vi "test缓存测试.vi"() -> ()   [LabVIEW 2017, in "时值缓存压缩模块.lvlib"]
panel:
  out "等级数量":cluster{i32[], "压缩等级数量":i32[]}(graph)
  out "真起始时间":timestamp
  out "实际缓存数量":i32
  in  "停止按钮":bool
  out "大小":i32
  out "缓存处理用时":dbl
  out "缓存数据":cluster{"时间":timestamp[], "数值":dbl[]}(graph)
  in  "等待时间（毫秒）":u32=500
  in  "容量限值":i32=300 min=1
  in  "变化基数":dbl=3.0
  in  "主值":dbl=25.0 format="%#_13g"
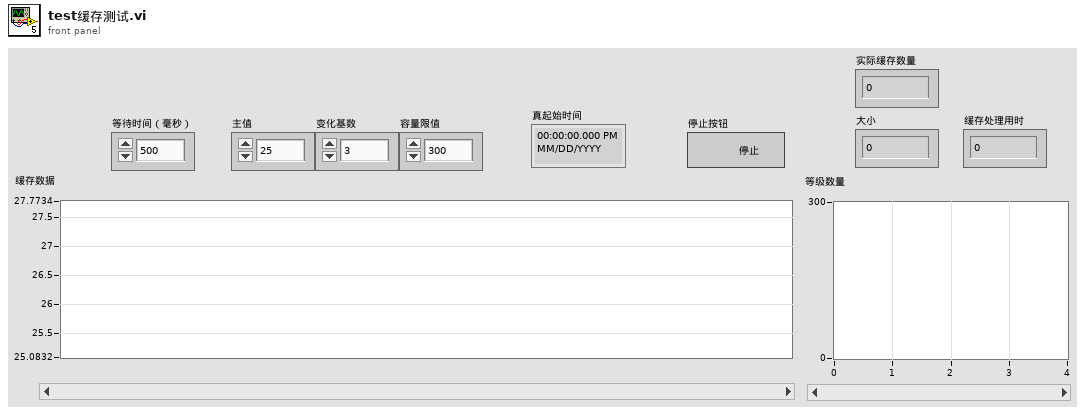
[diagram p1: front panel]
types:
  T1 = typedef "时值缓存压缩模块.lvlib/缓存数据.ctl" = cluster{"时间":timestamp[], "数值":dbl[], "压缩等级数量":i32[], "最大值":cluster{"时间":timestamp, "数值":dbl}, "起始点":cluster{"时间":timestamp, "数值":dbl}, "容量限值":i32, "报警累积":dbl}
  T2 = typedef "LVAnnotationListTypeDef.ctl" = cluster{"Name":string, "Color":u32, "Style":u8, "Point Style":u8, "Name Visible":bool, "Allow Drag":bool, "Annotation Mode":u32, "Plot":i32, "Index":i32, "Position":cluster{"X":dbl, "Y":dbl}, "X Scale":u32, "Y Scale":u32, "Show Arrow":bool, "Lock Name":bool, "Plot Area":i32, "Label Offset":cluster{"X":dbl, "Y":dbl}}[]
  T3 = cluster{"Name":string, "Color":u32, "Style":u8, "Point Style":u8, "Name Visible":bool, "Allow Drag":bool, "Annotation Mode":u32, "Plot":i32, "Index":i32, "Position":cluster{"X":dbl, "Y":dbl}, "X Scale":u32, "Y Scale":u32, "Show Arrow":bool, "Lock Name":bool, "Plot Area":i32, "Label Offset":cluster{"X":dbl, "Y":dbl}}
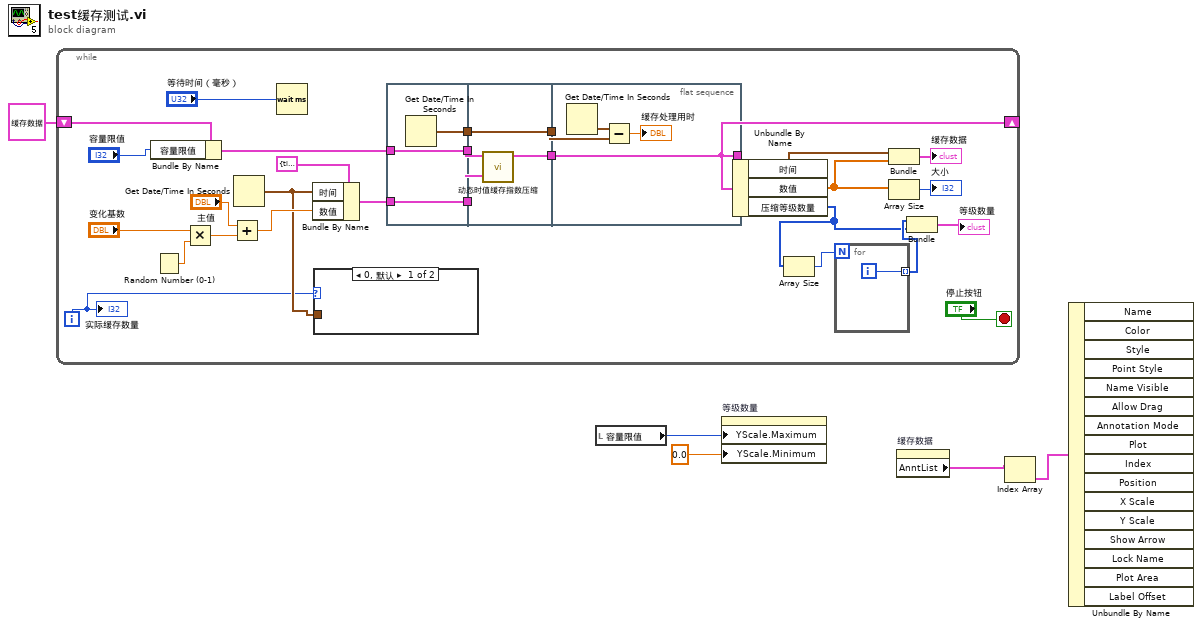
[diagram p0: block diagram]
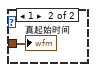
[diagram p2: hidden frame]
diagram:
  n1 = while {
    shift-right: [w22] -> _
    shift-left: T1 {"时间"=[], "数值"=[], "压缩等级数量"=[], "最大值"={"时间"=timestamp(0 s since 1904-01-01), "数值"=0.0}, "起始点"={"时间"=timestamp(0 s since 1904-01-01), "数值"=0.0}, "容量限值"=0, "报警累积"=0.0} ("缓存数据 i") -> [w26]
    i -> [w10]
    stop <- "停止按钮" stop-if-true
    n2 = Bundle By Name(cluster=w26, "容量限值"="容量限值") -> (w25:T1)
    n3 = Random Number (0-1)() -> (number: 0 to 1=w31:dbl)
    n4 = Multiply(x="变化基数", y=w31) -> (x*y=w32:dbl)
    n5 = Add(x="主值", y=w32) -> (x+y=w29:dbl)
    n6 = Get Date/Time In Seconds() -> (seconds since 1Jan1904=w11:timestamp)
    n7 = Wait (ms)(milliseconds to wait="等待时间（毫秒）") -> ()  [unwired: 1 out]
    n8 = Bundle By Name(cluster=cluster{"时间":timestamp, "数值":dbl} {"时间"=timestamp(0 s since 1904-01-01), "数值"=0.0} ("新数据"), "时间"=w11, "数值"=w29) -> (w27:cluster{"时间":timestamp, "数值":dbl})
    n9 = case shown="0, 默认" w10 {
      tunnel: w11 -> [_ w35]
      frame 0, Default {
      }
      frame 1 {
        "真起始时间" <- w35
      }
    }
    n10 = flat-sequence {
      tunnel: w25 -> [w37]
      tunnel: w27 -> [w38]
      tunnel: [w38] -> w19
      tunnel: [w37] -> w18
      tunnel: [w36] -> w16
      tunnel: w19 -> [w39]
      tunnel: w18 -> [w42]
      tunnel: [w41] -> w17
      tunnel: w16 -> [w40]
      tunnel: [w40] -> w15
      tunnel: [w46] -> w22
      tunnel: w17 -> [w46]
      tunnel: w15 -> [w44]
      frame #0 {
        n11 = Get Date/Time In Seconds() -> (seconds since 1Jan1904=w36:timestamp)
      }
      frame #1 {
        n12 = call "动态时值缓存指数压缩.vi"("新数据"=w39, "缓存数据"=w42) -> ("缓存数据 o"=w41:T1)  [unwired: 9 in]
      }
      frame #2 {
        n13 = Get Date/Time In Seconds() -> (seconds since 1Jan1904=w45:timestamp)
        n14 = Subtract(x=w45, y=w44) -> (x-y=→"缓存处理用时":dbl)
      }
    }
    n15 = Unbundle By Name(w22) -> ("时间"=w21:timestamp[], "数值"=w14:dbl[], "压缩等级数量"=w7:i32[])
    n16 = Array Size(array=w7) -> (size(s)=w9:i32)
    n17 = for {
      N: w9 -> [_]
      tunnel: [w34] -> w8 mode=indexing
      i -> [w34]
    }
    n18 = Bundle("时间"=w21, "数值"=w14) -> (→"缓存数据":cluster{"时间":timestamp[], "数值":dbl[]})  [unwired: 1 in]
    n19 = Array Size(array=w14) -> (size(s)=→"大小":i32)
    n20 = Bundle(w8, "压缩等级数量"=w7) -> (→"等级数量":cluster{i32[], "压缩等级数量":i32[]})  [unwired: 1 in]
    "实际缓存数量" <- w10
  }
  n21 = local read "容量限值"() -> (w1:i32)
  n22 = property on="等级数量" class="XYGraph (严格)"("YScale.Maximum"=w1, "YScale.Minimum"=0.0 ("Y标尺.范围:最小值")) -> ()  [unwired: 2 in, 2 out]
  n23 = property on="缓存数据" class="XYGraph (严格)"() -> ("AnntList"=w4:T2)  [unwired: 2 in, 2 out]
  n24 = Index Array(array=w4) -> (element=w3:T3)  [unwired: 1 in]
  n25 = Unbundle By Name(w3) -> ()  [unwired: 16 out]
